vi "Launch Single Assert Display.vi"(8 "error in (no error)":errorcluster, 10 "Assert UID":string, 11 "Main Display in":refnum<class "Main Display.lvclass">) -> (0 "error out":errorcluster, 3 "Main Display out":refnum<class "Main Display.lvclass">)   [LabVIEW 2016, in "Assert API Components.lvlib" / "Assert Display.lvlib" / "Main Display.lvlib" / "Main Display.lvclass"]
uses:
  Main Display.lvclass
  C:/Program Files (x86)/National Instruments/LabVIEW 2016/vi.lib/ActorFramework/Actor/Actor.lvclass
  Main Display.lvclass/Main Display.ctl
  Single Assert Display/Single Assert Display/Single Assert Display.lvclass
  <vilib>/ActorFramework/Actor/Actor.lvclass
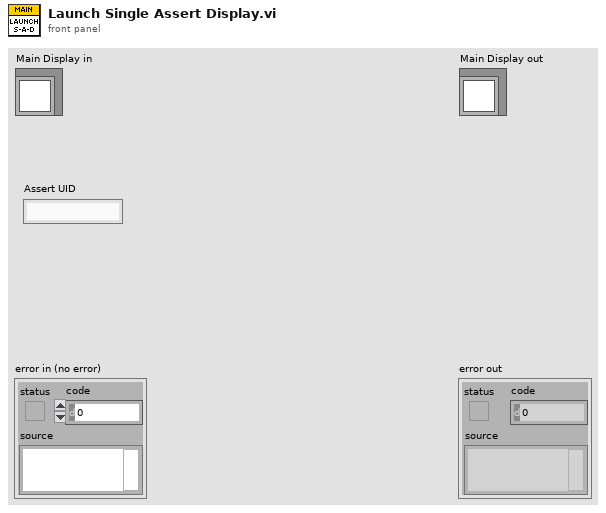
[diagram p1: front panel]
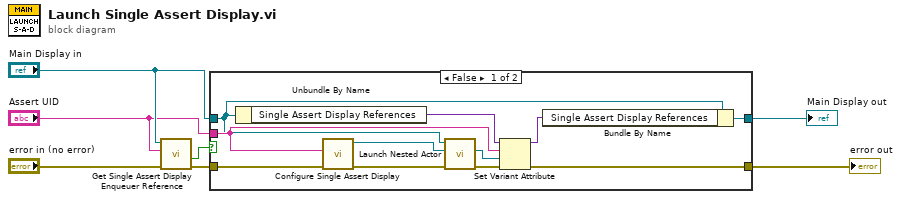
[diagram p0: block diagram]
diagram:
  n1 = call "Get Single Assert Display Enqueuer Reference.vi"("error in (no error)"="error in (no error)", "Assert UID"="Assert UID", "Main Display in"="Main Display in") -> ("error out"=w4:errorcluster, "Assert Display Active?"=w6:bool)  [unwired: 6 in, 1 out]
  n2 = case shown="False" w6 {
    tunnel: "Main Display in" -> [w11 w19]
    tunnel: w4 -> [w16 w20]
    tunnel: "Assert UID" -> [w14 _]
    tunnel: [w9 w20] -> w2
    tunnel: [w8 w19] -> w1
    frame False {
      n3 = Unbundle By Name(w11) -> ("Single Assert Display References"=w15:variant)
      n4 = call "Configure Single Assert Display.vi"("error in (no error)"=w16, "Assert UID"=w14) -> ("error out"=w17:errorcluster, "Single Assert Display out"=w18:refnum<class "Single Assert Display.lvclass">)  [unwired: 8 in]
      n5 = call <vilib>:"Launch Nested Actor.vi"("error in (no error)"=w17, "Nested Actor"=w18, "Caller Actor in"=w11) -> ("error out"=w12:errorcluster, "Nested Actor's Enqueuer"=w13:refnum<class "Message Enqueuer.lvclass">)  [unwired: 6 in, 1 out]
      n6 = Set Variant Attribute(Variant=w15, name=w14, value=w13, error in=w12) -> (Variant out=w10:variant, error out=w9:errorcluster)  [unwired: 1 out]
      n7 = Bundle By Name(cluster=w11, "Single Assert Display References"=w10) -> (w8:refnum<class "Main Display.lvclass">)
    }
    frame True {
    }
  }
  "error out" <- w2
  "Main Display out" <- w1
